vi "Cond Attr Create Object.vi"(8 "error in (no error)":errorcluster, 11 "cond attr pointer in":u64) -> (0 "error out":errorcluster, 3 "Cond Attr out":T1)   [LabVIEW 2013, in "Linux RT IPC.lvlib" / "POSIX Threads.lvlib" / "Cond Attr.lvclass"]
doc: "Creates a LabVIEW object used to encapsulate a pthread cond attribute object referenced by cond attr pointer."
uses:
  Cond Attr.lvclass
  Controls/reference.ctl
  POSIX Thread Object/POSIX Thread Object.lvclass/POSIX Thread Object.ctl
  POSIX Thread Object/POSIX Thread Object.lvclass
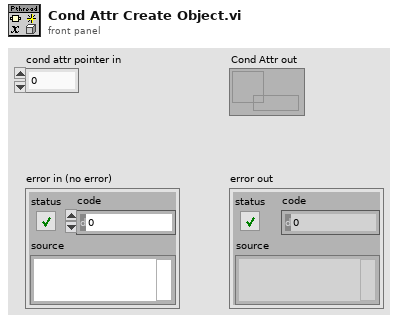
[diagram p1: front panel]
types:
  T1 = typedef "Linux RT IPC.lvlib/POSIX Threads.lvlib/Cond Attr.lvclass/reference.ctl" = refnum<data-value>
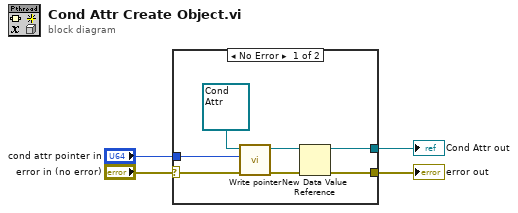
[diagram p0: block diagram]
diagram:
  n1 = case shown="No Error" "error in (no error)" {
    selector: "error in (no error)" -> [w8 w12]
    tunnel: "cond attr pointer in" -> [w9 _]
    tunnel: [w7 w12] -> w2
    tunnel: [w6 _] -> w1
    frame No Error {
      n2 = call "Write pointer.vi"("error in (no error)"=w8, "pointer"=w9, "POSIX Thread Object in"=refnum<class "Cond Attr.lvclass"> refnum ("POSIX Threads.lvlib:Cond.lvclass")) -> ("error out"=w10:errorcluster, "POSIX Thread Object out"=w11:refnum<class "Cond Attr.lvclass">)  [unwired: 7 in]
      n3 = New Data Value Reference(data value=w11, error in=w10) -> (data value reference=w6:refnum<data-value>, error out=w7:errorcluster)
    }
    frame Error {
    }
  }
  "Cond Attr out" <- w1
  "error out" <- w2
